vi "sub_hw-check.vi"(11 "GNSS str":string) -> (3 "val":bool)   [LabVIEW 2019]
panel:
  out "ubx val":bool
  out "nmea val":bool
  out "u8arr":u8[](array[numeric])=[242, 168, 144, 180, 0, 0, 0, 31, 156, 89, 53, 19, 184, 201, 131, 170, 128, 138, 2, 240, 31, 128, 31, 4, 6, 5, 119, 186, 39, 29, 138, 100, 165, 88, 13, 227, 116, 5, 38, 132, 118, 58, 63, 131, 40, 38, 105, 27, 134, 8, 178, 43, 61, 225, 200, 73, 1, 143, 51, 93, 247, 184, 93, 204, 170, 65, 192, 7, 32, 231, 62, 64, 196, 98, 1, 163, 215, 33, 136, 178, 224, 172, 114, 112, 204, 51, 12, 195, 44, 132, 51, 12, 158, 14, 8, 0, 2, 220, 24, 5, 129, 96, 58, 22, 134, 32, 240, 84, 13, 0, 108, 224, 218, 39, 122, 79, 15, 37, 156, 48, 70, 95, 148, 66, 81, 173, 140, 253, 160, 0, 0, 0, 0, 0, 0, 0, 0, 0, 0, 0, 0, 0, 0, 0, 0, 0, 0, 0, 0, 0, 0, 0, 0, 0, 0, 0, 0, 0, 0, 0, 0, 0, 0, 0, 0, 0, 0, 0, 0, 109, 131, 114, 211, 0, 8, 76, 224, 0, 138, 0, 0, 0, 0, 168, 247, 42, 211, 0, 62, 254, 128, 1, 0, 0, 0, 20, 28, 69, 14, 0, 0, 0, 8, 0, 0, 0, 0, 0, 0, 0, 1, 253, 143, 0, 7, 2, 0, 252, 24, 0, 14, 2, 3, 250, 121, 0, 23, 5, 0, 0, 0, 0, 0, 5, 1, 252, 84, 0, 252, 6, 0, 253, 242, 0, 6, 6, 1, 253, 45, 0, 19, 193, 101, 164, 181, 98, 1, 7, 92, 0, 56, 20, 113, 16, 228, 7, 12, 30, 4, 37, 8, 55, 2, 0, 0, 0, 170, 39, 232, 11, 3, 1, 234, 22, 101, 215, 170, 75, 230, 233, 73, 22, 115, 252, 0, 0, 64, 180, 0, 0, 90, 2, 0, 0, 229, 2, 0, 0, 242, 255, 255, 255, 5, 0, 0, 0, 231, 255, 255, 255, 14, 0, 0, 0, 0, 0, 0, 0, 132, 0, 0, 0, 252, 187, 229, 0, 117, 0, 0, 0, 186, 101, 67, 44, 0, 0, 0, 0, 0, 0, 0, 0, 134, 196, 181, 98, 1, 59, 40, 0, 0, 0, 0, 0, 56, 20, 113, 16, 0, 0, 0, 0, 0, 0, 0, 0, 0, 0, 0, 0, 0, 0, 0, 0, 0, 0, 0, 0, 0, 0, 0, 0, 0, 0, 0, 0, 0, 0, 0, 0, 49, 83, 211, 0, 126, 254, 128, 0, 1, 0, 0, 20, 28, 69, 14, 0, 7, 28, 198, 225, 30, 4, 184, 99, 125, 118, 145, 240, 72, 226, 103, 255, 254, 104, 0, 1, 136, 0, 0, 85, 255, 255, 252, 88, 0, 0, 0, 100, 0, 0, 1, 6, 142, 40, 127, 255, 255, 210, 111, 74, 223, 255, 255, 254, 108, 189, 176, 0, 0, 4, 49, 170, 104, 0, 0, 0, 84, 93, 246, 0, 0, 0, 41, 3, 184, 0, 0, 0, 5, 38, 23, 255, 255, 255, 252, 168, 113, 0, 0, 0, 4, 100, 194, 0, 0, 0, 42, 241, 206, 0, 0, 0, 2, 163, 136, 0, 0, 0, 115, 231, 144, 0, 0, 173, 240, 0, 0, 31, 40, 0, 0, 156, 233, 191, 36, 71, 78, 71, 71, 65, 44, 48, 52, 51, 55, 48, 56, 46, 50, 48, 44, 51, 55, 50, 51, 46, 54, 53, 54, 53, 53, 44, 78, 44, 49, 50, 54, 53, 54, 46, 57, 50, 52, 55, 55, 44, 69, 44, 49, 44, 49, 50, 44, 48, 46, 54, 57, 44, 52, 54, 46, 49, 44, 77, 44, 49, 56, 46, 53, 44, 77, 44, 44, 42, 55, 50, 13, 10] format="%02x"
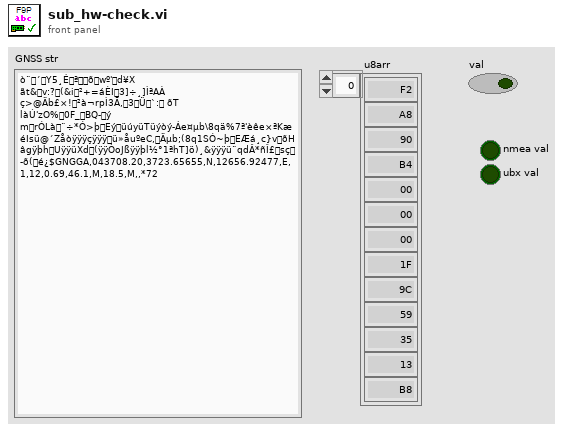
[diagram p1: front panel]
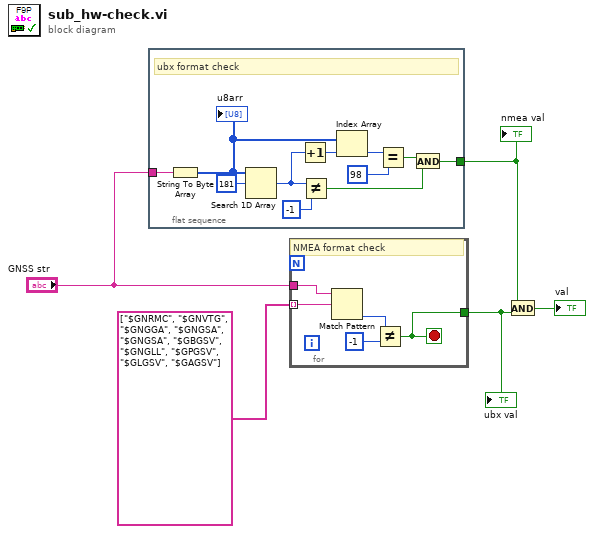
[diagram p0: block diagram]
diagram:
  n1 = flat-sequence {
    tunnel: "GNSS str" -> [w16]
    tunnel: [w6] -> w2
    frame #0 {
      # "ubx format check"
      n2 = String To Byte Array(string=w16) -> (unsigned byte array=w14:u8[])
      "u8arr" <- w14
      n3 = Search 1D Array(1D array=w14, element=u8 181 ("원소")) -> (index of element=w12:i32)  [unwired: 1 in]
      n4 = Increment(x=w12) -> (x+1=w13:i32)
      n5 = Not Equal?(x=w12, y=-1) -> (x != y?=w7:bool)
      n6 = Index Array(array=w14, index=w13) -> (element=w10:u8)
      n7 = Equal?(x=w10, y=u8 98) -> (x = y?=w8:bool)
      n8 = And(x=w8, y=w7) -> (x .and. y?=w6:bool)
    }
  }
  n9 = for {
    tunnel: string[] ["$GNRMC", "$GNVTG", "$GNGGA", "$GNGSA", "$GNGSA", "$GBGSV", "$GNGLL", "$GPGSV", "$GLGSV", "$GAGSV"] ("배열") -> [w19] mode=indexing
    tunnel: [w20] -> w1
    tunnel: "GNSS str" -> [w18]
    stop <- w20 stop-if-true
    # "NMEA format check"
    n10 = Match Pattern(string=w18, regular expression=w19) -> (offset past match=w17:i32)  [unwired: 1 in, 3 out]
    n11 = Not Equal?(x=w17, y=-1) -> (x != y?=w20:bool)
  }
  "ubx val" <- w1
  n12 = And(x=w2, y=w1) -> (x .and. y?=→"val":bool)
  "nmea val" <- w2
